vi "String to Bool.vi"(8 "error in":errorcluster, 11 "Integer String":string) -> (0 "error out":errorcluster, 3 "Bool":bool)   [LabVIEW 2020, in "CANopen.lvlib"]
doc: "A string that contains the number to convert."
uses:
  CANopen.lvlib
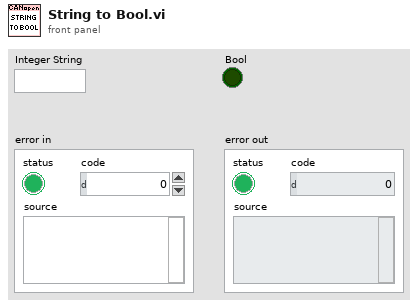
[diagram p1: front panel]
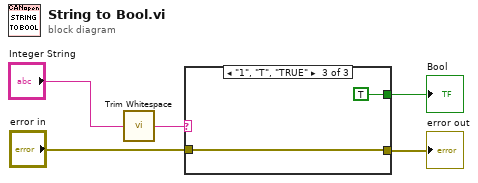
[diagram p0: block diagram]
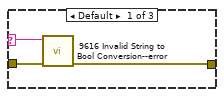
[diagram p2: hidden frame]
diagram:
  n1 = call <vilib>:"Trim Whitespace.vi"("string"="Integer String") -> ("trimmed string"=w1:string)  [unwired: 1 in]
  n2 = case shown="\"1\", \"T\", \"TRUE\"" w1 {
    selector: w1 -> [w6 _ _]
    tunnel: [w7 w9 w10] -> w5
    tunnel: "error in" -> [w8 w9 w10]
    tunnel: [_ _ TRUE] -> w2
    frame Default {
      n3 = call "9616 Invalid String to Bool Conversion--error.vi"("error in"=w8, "Argument"=w6) -> ("error out"=w7:errorcluster)  [unwired: 9 in]
    }
    frame "0", "F", "FALSE" {
    }
    frame "1", "T", "TRUE" {
    }
  }
  "Bool" <- w2
  "error out" <- w5
